vi "DAQ@Filter__Parameter.vi"(1 "ParamterIn":string) -> (0 "ParamterOut":string)   [LabVIEW 2019]
panel:
  in  "ParameterS":string(combo)
  in  "FilterType":string(combo)
  in  "WaveFormName":string(combo)
  in  "Confirm":bool
  # "DAQ@Filter $WaveForm,$Filter,$ParameterS...............\n------------------------------------------------------------------------------------------------------------------------------------------\nMOVINGAVERAGE    $WaveForm,MOVINGAVERAGE{,number of points}"
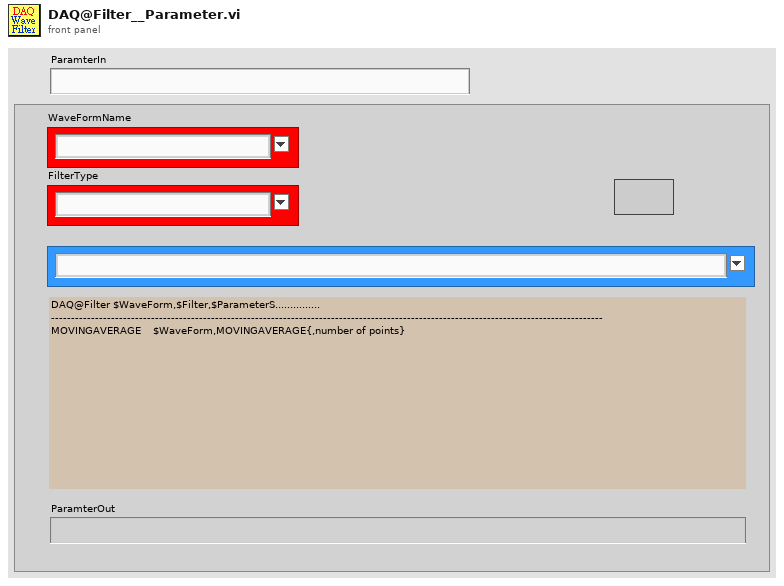
[diagram p1: front panel]
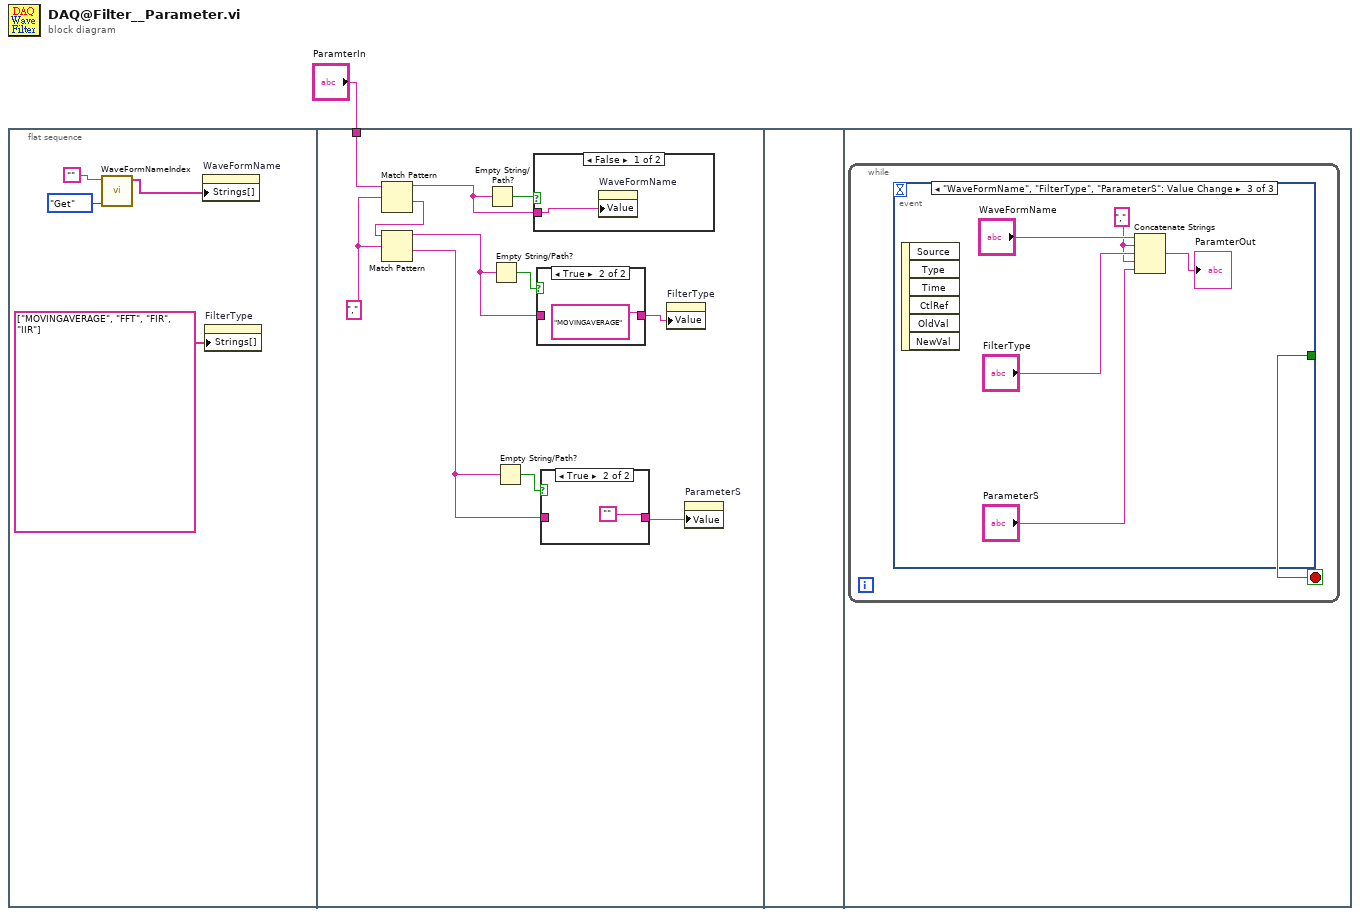
[diagram p0: block diagram]
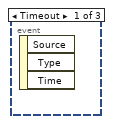
[diagram p5: hidden frame]
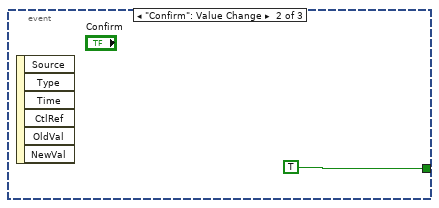
[diagram p6: hidden frame]
diagram:
  n1 = flat-sequence {
    tunnel: "ParamterIn" -> [w11]
    frame #0 {
      n2 = call "WaveFormNameIndex.vi"("OP"=enum16{"Get", "Update", "Init", "GetSPS"}."Get", "WaveFormName"="") -> ("WaveFormNameList"=w2:string[])  [unwired: 6 in, 3 out]
      n3 = property on="WaveFormName" class="CmbBox"("Strings[]"=w2) -> ()  [unwired: 2 in, 2 out]
      n4 = property on="FilterType" class="CmbBox"("Strings[]"=string[] ["MOVINGAVERAGE", "FFT", "FIR", "IIR"] ("Strings []")) -> ()  [unwired: 2 in, 2 out]
    }
    frame #1 {
      w7 = "," ("search string/char (-)")
      n5 = Match Pattern(string=w11, regular expression=w7) -> (before substring=w10:string, after substring=w9:string)  [unwired: 1 in, 2 out]
      n6 = Match Pattern(string=w9, regular expression=w7) -> (before substring=w8:string, after substring=w6:string)  [unwired: 1 in, 2 out]
      n7 = Empty String/Path?(string/path=w10) -> (empty?=w16:bool)
      n8 = Empty String/Path?(string/path=w8) -> (empty?=w15:bool)
      n9 = Empty String/Path?(string/path=w6) -> (empty?=w13:bool)
      n10 = case shown="False" w16 {
        tunnel: w10 -> [w21 _]
        frame False {
          n11 = property on="WaveFormName" class="CmbBox"("Value"=w21) -> ()  [unwired: 2 in, 2 out]
        }
        frame True {
        }
      }
      n12 = case shown="True" w15 {
        tunnel: [w19 "MOVINGAVERAGE"] -> w14
        tunnel: w8 -> [w19 _]
        frame False {
        }
        frame True {
        }
      }
      n13 = case shown="True" w13 {
        tunnel: [w17 ""] -> w12
        tunnel: w6 -> [w17 _]
        frame False {
        }
        frame True {
        }
      }
      n14 = property on="FilterType" class="CmbBox"("Value"=w14) -> ()  [unwired: 2 in, 2 out]
      n15 = property on="ParameterS" class="CmbBox"("Value"=w12) -> ()  [unwired: 2 in, 2 out]
    }
    frame #2 {
    }
    frame #3 {
      n16 = while {
        stop <- w22 stop-if-true
        n17 = event shown="[2] \"WaveFormName\", \"FilterType\", \"ParameterS\": Value Change" {
          selector: _ -> [_ _ _]
          dyn-events: _ -> [_ _ _]
          timeout: _ -> [_ _ _]
          tunnel: [_ TRUE _] -> w22
          event Timeout {
            n18 = event-data() -> ()  [unwired: 1 in, 3 out]
          }
          event "Confirm": Value Change {
            n19 = event-data() -> ()  [unwired: 1 in, 6 out]
          }
          event "WaveFormName", "FilterType", "ParameterS": Value Change {
            w25 = ","
            n20 = event-data() -> ()  [unwired: 1 in, 6 out]
            n21 = Concatenate Strings("WaveFormName", w25, "FilterType", w25, "ParameterS") -> (→"ParamterOut":string)
          }
        }
      }
    }
  }
